vi "Write current stack.vi"(8 "error in (no error)":errorcluster, 9 "Current stack":u16, 10 "File name":path, 11 "Tomo in":refnum<class "Tomo.lvclass">) -> (0 "error out":errorcluster, 3 "Tomo out":refnum<class "Tomo.lvclass">)   [LabVIEW 2012, in "Tomo.lvclass"]
uses:
  Tomo.lvclass
  <vilib>/Utility/file.llb/Write To Spreadsheet File (DBL).vi
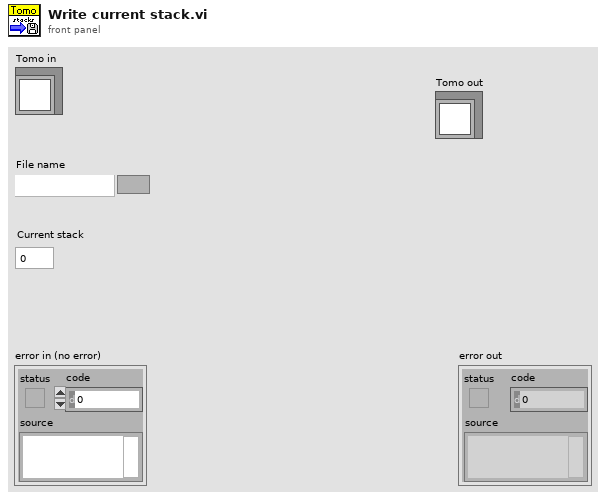
[diagram p1: front panel]
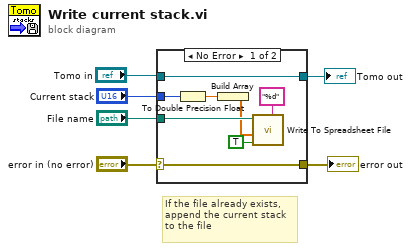
[diagram p0: block diagram]
diagram:
  # "If the file already exists,\nappend the current stack\nto the file"
  n1 = case shown="No Error" "error in (no error)" {
    selector: "error in (no error)" -> [w14 w16]
    tunnel: [w14 w16] -> w5
    tunnel: [w12 w15] -> w1
    tunnel: "Tomo in" -> [w12 w15]
    tunnel: "File name" -> [w13 _]
    tunnel: "Current stack" -> [w7 _]
    frame No Error {
      n2 = To Double Precision Float(number=w7) -> (double precision float=w10:dbl)
      n3 = Build Array(w10) -> (w11:dbl[])
      n4 = call-poly <vilib>:"Write To Spreadsheet File.vi"("format (%.3f)"="%d", "append to file? (new file:F)"=TRUE, "1D data"=w11, "file path (dialog if empty)"=w13) -> ()  [unwired: 4 in, 1 out]
    }
    frame Error {
    }
  }
  "error out" <- w5
  "Tomo out" <- w1
